vi "Stop Core.vi"(10 "final error code":i32, 11 "Calculadora in":refnum<class "Calculadora.lvclass">) -> (3 "Calculadora out":refnum<class "Calculadora.lvclass">)   [LabVIEW 2020, in "Calculadora.lvlib" / "Calculadora.lvclass"]
doc: "(<B>Filename</B>: Actor Framework.lvlib:Actor.lvclass:Stop Core.vi)\n\nDefines what the actor does before it stops. Use the <B>final error code</B> input to determine whether the actor shut down in response to an error.\n\nBy default, this method passes the Stop message along to all auto-stop nested actors. A descendant class may override this method to define additional behavior, such as shutting down any processes the actor initiated in its override of the Actor Core method."
uses:
  Calculadora.lvclass
  Calculadora.lvclass/Calculadora.ctl
  <vilib>/ActorFramework/Actor/Actor.lvclass
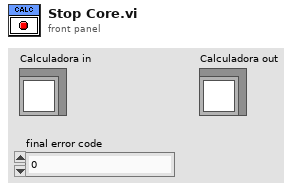
[diagram p1: front panel]
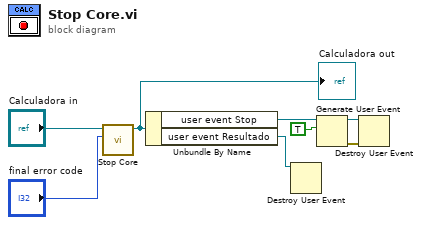
[diagram p0: block diagram]
diagram:
  n1 = call-parent "Stop Core.vi"("final error code"="final error code", "Actor in"="Calculadora in") -> ("Actor out"=w6:refnum<class "Calculadora.lvclass">)  [unwired: 9 in]
  "Calculadora out" <- w6
  n2 = Unbundle By Name(w6) -> ("user event Stop"=w5:refnum<user-event>, "user event Resultado"=w1:refnum<user-event>)
  n3 = Destroy User Event(user event=w1) -> ()  [unwired: 1 in, 1 out]
  n4 = Generate User Event(user event=w5, event data cluster=TRUE ("event data")) -> (user event out=w3:refnum<user-event>, error out=w2:errorcluster)  [unwired: 2 in]
  n5 = Destroy User Event(user event=w3, error in=w2) -> ()  [unwired: 1 out]
